vi "Begin.vi"(11 "Image Size":T1=enum."160x120") -> (0 "error out":errorcluster)   [LabVIEW 2011]
doc: "Called before other user functions, this VI is expected to open initial I/O refnums, load in file data, and do all program initialization. Notice that the <B>error out</B> terminal is simply used for data flow. Wiring it to other structures or subVIs ensures that this VI runs first."
uses:
  <vilib>/Rock Robotics/WPI/Camera/WPI_CameraImageSize.ctl
  <vilib>/Rock Robotics/WPI/Joystick/WPI_JoystickDeviceEnum.ctl
  <vilib>/Rock Robotics/WPI/Camera/WPI_CameraWhite Balance Values.ctl
  <vilib>/Rock Robotics/WPI/Camera/WPI_CameraExposure Values.ctl
  <vilib>/Rock Robotics/WPI/Camera/WPI_CameraFrameRate.ctl
  <vilib>/Rock Robotics/SystemInterfaces/DIO/FPGA_DIOPWMChannel.ctl
  <vilib>/Rock Robotics/SystemInterfaces/AI/FPGA_AIChannel.ctl
  <vilib>/Rock Robotics/WPI/MotorControl/WPI_MotorControlOpen Victor.vi
  Robot Global Data.vi
  <vilib>/Rock Robotics/WPI/RobotDrive/WPI_RobotDriveOpen4MotorWithJaguar.vi
  <vilib>/Rock Robotics/WPI/RobotDrive/WPI_RobotDriveOpen2MotorWithCANJaguar.vi
  <vilib>/Rock Robotics/WPI/RobotDrive/WPI_RobotDriveOpen4MotorWithCANJaguar.vi
  <vilib>/Rock Robotics/WPI/RobotDrive/WPI_RobotDriveOpen2MotorWithJaguar.vi
panel:
  in  "4 Moter":bool
  in  "Enable CAN":bool=TRUE
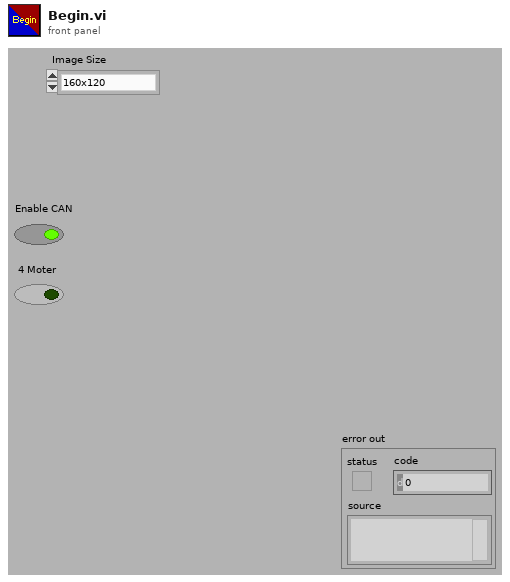
[diagram p1: front panel]
types:
  T1 = typedef "WPI_CameraImageSize.ctl" = enum16{"640x480", "320x240", "160x120"}
  T2 = typedef "FPGA_DIOPWMChannel.ctl" = enum8{"PWM 1", "PWM 2", "PWM 3", "PWM 4", "PWM 5", "PWM 6", "PWM 7", "PWM 8", "PWM 9", "PWM 10", "Invalid"}
  T3 = typedef "FPGA_AIChannel.ctl" = enum8{"AI 1", "AI 2", "AI 3", "AI 4", "AI 5", "AI 6", "AI 7", "AI 8", "Invalid"}
  T4 = typedef "WPI_JoystickDeviceEnum.ctl" = enum16{"USB 1", "USB 2", "USB 3", "USB 4", "Kinect 1", "Kinect 2"}
  T5 = typedef "WPI_CameraFrameRate.ctl" = u32
  T6 = typedef "WPI_CameraExposure Values.ctl" = enum16{"Auto", "Flicker-free 50 Hz", "Flicker-free 60 Hz", "Hold current"}
  T7 = typedef "WPI_CameraWhite Balance Values.ctl" = enum16{"Auto", "Fixed indoor", "Fixed outdoor 1", "Fixed outdoor 2", "Fixed fluorescent 1", "Fixed fluorescent 2", "Hold current"}
  T8 = typedef "WPI_JoystickDevRef.ctl" = cluster{"Device":T4}
  T9 = typedef "WPI_RobotDriveDevRef.ctl" = cluster{"DevStatus":errorcluster, "Motors[]":T10[], "Square Inputs":bool, "Max Output":dbl, "Isochronous":bool}
  T10 = typedef "WPI_MotorControlDeviceRef.ctl" = cluster{"DeviceStatus":errorcluster, "Type":enum16{"PWM", "CAN"}, "PWM":cluster{"Digital Module":T11, "PWM Channel":T2, "DeadBand":T12}, "CAN":cluster{"Device Number":u8, "Control Mode":T13, "Semaphore":T14, "Max Vout":dbl}, "Invert":bool, "TransformRef":T15, "InvTransformRef":T15}
  T11 = typedef "FPGA_TypedefDigitalModule.ctl" = enum16{"Digital Module 1", "Digital Module 2"}
  T12 = typedef "WPI_PWMDeadband.ctl" = cluster{"Name":string, "maxPositivePwm":i32, "minPositivePwm":i32, "centerPwm":i32, "maxNegativePwm":i32, "minNegativePwm":i32, "angularRange":u16}
  T13 = typedef "WPI_CANJaguar_ControlMode.ctl" = enum8{"Percent VBus", "Current", "Speed", "Position", "Voltage"}
  T14 = typedef "Semaphore RefNum" = refnum<k1>
  T15 = typedef "WPI_PWMTransform_ConPane.ctl" = refnum<vi>
  T16 = typedef "WPI_JoystickButtonState.ctl" = cluster{"Button 1":bool, "Button 2":bool, "Button 3":bool, "Button 4":bool, "Button 5":bool, "Button 6":bool, "Button 7":bool, "Button 8":bool, "Button 9":bool, "Button 10":bool, "Button 11":bool, "Button 12":bool}
  T17 = typedef "WPI_CameraDevRef.ctl" = cluster{"Camera Address":string, "CameraStatus":errorcluster, "Acquire Image Notifier":refnum<notifier>}
  T18 = enum16{"CAN Bcast - don't use", "CAN Defualt - don't use", "CAN 2 - Black Jag", "CAN 3", "CAN 4", "CAN 5", "CAN 6", "CAN 7", "CAN 8", "CAN 9"}
  T19 = typedef "WPI_AnalogChannelDevRef.ctl" = cluster{"DevStatus":errorcluster, "Analog Module":T20, "Analog Channel":T3}
  T20 = typedef "FPGA_TypedefAnalogModule.ctl" = enum16{"Analog Module 1", "Analog Module 2"}
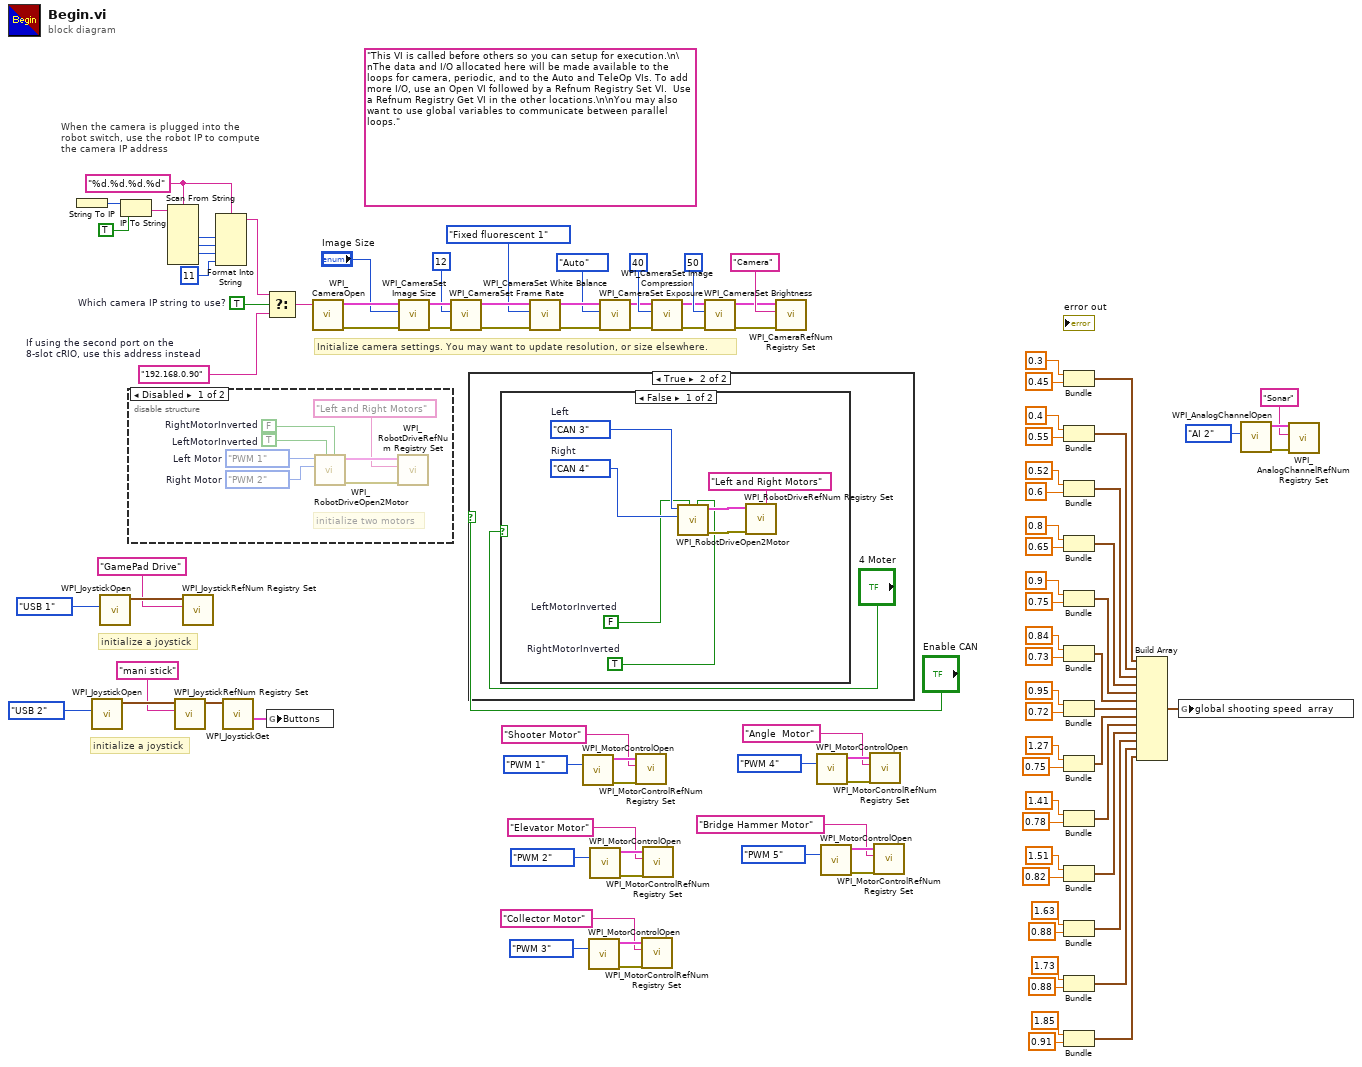
[diagram p0: block diagram]
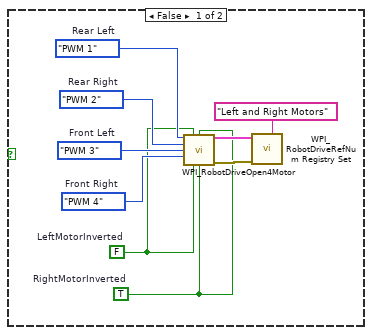
[diagram p2: hidden frame]
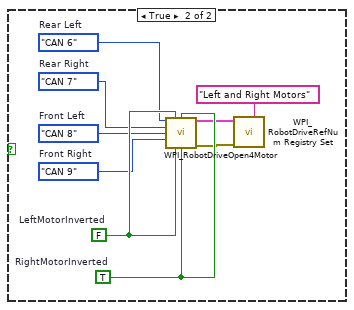
[diagram p3: hidden frame]
diagram:
  w71 = TRUE  # Which camera IP string to use?
  w75 = "%d.%d.%d.%d" ("format string")
  (unwired) "This VI is called before others so you can setup for execution.\n\nThe data and I/O allocated here will be made available to the loops for camera, periodic, and to the Auto and TeleOp VIs. To add more I/O, use an Open VI followed by a Refnum Registry Set VI.  Use a Refnum Registry Get VI in the other locations.\n\nYou may also want to use global variables to communicate between parallel loops."
  w72 = "192.168.0.90"  # If using the second port on the 8-slot cRIO, use this address instead
  # "initialize a joystick"
  # "When the camera is plugged into the\nrobot switch, use the robot IP to compute\nthe camera IP address"
  # "initialize a joystick"
  # "Initialize camera settings. You may want to update resolution, or size elsewhere."
  n1 = String To IP() -> (0:w82:u32)  [unwired: 1 in]
  n2 = call <vilib>:"WPI_JoystickOpen.vi"("JoystickDevice"=WPI_JoystickDeviceEnum."USB 2") -> ("JoystickDevRef"=w65:T8)  [unwired: 10 out]
  n3 = call <vilib>:"WPI_JoystickOpen.vi"("JoystickDevice"=WPI_JoystickDeviceEnum."USB 1") -> ("JoystickDevRef"=w105:T8)  [unwired: 10 out]
  n4 = IP To String(1:TRUE ("dot notation? (F)"), 2:w82) -> (0:w80:string)
  n5 = disable-structure shown="Disabled" {
    frame Disabled {
      w107 = FPGA_DIOPWMChannel."PWM 2"  # Right Motor
      w108 = FPGA_DIOPWMChannel."PWM 1"  # Left Motor
      w112 = TRUE  # LeftMotorInverted
      w113 = FALSE  # RightMotorInverted
      # "initialize two motors"
      n6 = call-poly <vilib>:"WPI_RobotDriveOpen2Motor.vi"("Right Motor Inverted"=w113, "Left Motor Inverted"=w112, "Right Motor"=w107, "Left Motor"=w108) -> ("error out"=w109:errorcluster, "RobotDriveDevRef"=w111:T9)  [unwired: 1 in, 5 out]
      n7 = call <vilib>:"WPI_RobotDriveRefNum Registry Set.vi"("error in (no error)"=w109, "refnum name"="Left and Right Motors", "RobotDriveDevRef"=w111) -> ()  [unwired: 9 out]
    }
    frame Enabled {
    }
  }
  n8 = Scan From String(format string=w75, input string=w80) -> (output 1=w79:i32, output 2=w78:i32, output 3=w77:i32)  [unwired: 7 in, 3 out]
  n9 = call <vilib>:"WPI_JoystickRefNum Registry Set.vi"("refnum name"="mani stick", "JoystickDevRef"=w65) -> ("JoystickDevRef"=w58:T8)  [unwired: 1 in, 8 out]
  n10 = call <vilib>:"WPI_JoystickRefNum Registry Set.vi"("refnum name"="GamePad Drive", "JoystickDevRef"=w105) -> ()  [unwired: 1 in, 9 out]
  n11 = Format Into String(format string=w75, w79, w78, w77, 11 ("Compression")) -> (resulting string=w73:string)  [unwired: 2 in, 1 out]
  n12 = call <vilib>:"WPI_JoystickGet.vi"("JoystickDevRef"=w58) -> ("Buttons"=w57:T16)  [unwired: 4 in, 2 out]
  n13 = Select(t=w73, s=w71, f=w72) -> (s? t:f=w74:string)
  n14 = global write "Robot Global Data.vi" "Buttons"(w57) -> ()
  n15 = call <vilib>:"WPI_CameraOpen.vi"("Camera Address"=w74) -> ("error out"=w95:errorcluster, "CameraDevRef"=w96:T17)  [unwired: 1 in, 8 out]
  n16 = call <vilib>:"WPI_CameraSet Image Size.vi"("error in (no error)"=w95, "Image Size"="Image Size", "CameraDevRef"=w96) -> ("error out"=w94:errorcluster, "CameraDevRef Out"=w97:T17)  [unwired: 7 out]
  n17 = call <vilib>:"WPI_CameraSet Frame Rate.vi"("error in (no error)"=w94, "Frame Rate (fps)"=T5 12, "CameraDevRef"=w97) -> ("error out"=w93:errorcluster, "CameraDevRef Out"=w99:T17)  [unwired: 7 out]
  n18 = case shown="True" "Enable CAN" {
    frame False {
      w116 = FPGA_DIOPWMChannel."PWM 4"  # Front Right
      w117 = FPGA_DIOPWMChannel."PWM 3"  # Front Left
      w118 = FPGA_DIOPWMChannel."PWM 2"  # Rear Right
      w119 = FPGA_DIOPWMChannel."PWM 1"  # Rear Left
      w115 = FALSE  # LeftMotorInverted
      w114 = TRUE  # RightMotorInverted
      n19 = call-poly <vilib>:"WPI_RobotDriveOpen4Motor.vi"("Rear Left Motor"=w119, "Rear Left Motor Inverted"=w115, "Rear Right Motor Inverted"=w114, "Rear Right Motor"=w118, "Front Left Motor"=w117, "Front Right Motor"=w116, "Front Left Motor Inverted"=w115, "Front Right Motor Inverted"=w114) -> ("RobotDriveDevRef"=w122:T9, "error out"=w120:errorcluster)  [unwired: 1 in, 5 out]
      n20 = call <vilib>:"WPI_RobotDriveRefNum Registry Set.vi"("error in (no error)"=w120, "refnum name"="Left and Right Motors", "RobotDriveDevRef"=w122) -> ()  [unwired: 9 out]
    }
    frame True {
      n21 = case shown="False" "4 Moter" {
        frame False {
          w126 = T18."CAN 4"  # Right
          w127 = T18."CAN 3"  # Left
          w125 = FALSE  # LeftMotorInverted
          w124 = TRUE  # RightMotorInverted
          n22 = call-poly <vilib>:"WPI_RobotDriveOpen2Motor.vi"("Right Motor Inverted"=w124, "Left Motor Inverted"=w125, "Right Motor"=w126, "Left Motor"=w127) -> ("error out"=w130:errorcluster, "RobotDriveDevRef"=w128:T9)  [unwired: 6 in]
          n23 = call <vilib>:"WPI_RobotDriveRefNum Registry Set.vi"("error in (no error)"=w130, "refnum name"="Left and Right Motors", "RobotDriveDevRef"=w128) -> ()  [unwired: 9 out]
        }
        frame True {
          w131 = T18."CAN 9"  # Front Right
          w132 = T18."CAN 8"  # Front Left
          w133 = T18."CAN 7"  # Rear Right
          w134 = T18."CAN 6"  # Rear Left
          w138 = FALSE  # LeftMotorInverted
          w139 = TRUE  # RightMotorInverted
          n24 = call-poly <vilib>:"WPI_RobotDriveOpen4Motor.vi"("Rear Left Motor"=w134, "Rear Left Motor Inverted"=w138, "Rear Right Motor Inverted"=w139, "Rear Right Motor"=w133, "Front Left Motor"=w132, "Front Right Motor"=w131, "Front Left Motor Inverted"=w138, "Front Right Motor Inverted"=w139) -> ("RobotDriveDevRef"=w135:T9, "error out"=w137:errorcluster)  [unwired: 1 in, 5 out]
          n25 = call <vilib>:"WPI_RobotDriveRefNum Registry Set.vi"("error in (no error)"=w137, "refnum name"="Left and Right Motors", "RobotDriveDevRef"=w135) -> ()  [unwired: 9 out]
        }
      }
    }
  }
  n26 = call <vilib>:"WPI_CameraSet White Balance.vi"("error in (no error)"=w93, "White Balance"=WPI_CameraWhite_Balance_Values."Fixed fluorescent 1", "CameraDevRef"=w99) -> ("error out"=w92:errorcluster, "CameraDevRef Out"=w98:T17)  [unwired: 7 out]
  n27 = call-poly <vilib>:"WPI_MotorControlOpen.vi"("PWM Channel"=FPGA_DIOPWMChannel."PWM 1") -> ("error out"=w69:errorcluster, "MotorControlDeviceRef"=w68:T10)  [unwired: 9 in]
  n28 = call-poly <vilib>:"WPI_MotorControlOpen.vi"("PWM Channel"=FPGA_DIOPWMChannel."PWM 3") -> ("error out"=w12:errorcluster, "MotorControlDeviceRef"=w11:T10)  [unwired: 9 in]
  n29 = call-poly <vilib>:"WPI_MotorControlOpen.vi"("PWM Channel"=FPGA_DIOPWMChannel."PWM 2") -> ("error out"=w16:errorcluster, "MotorControlDeviceRef"=w15:T10)  [unwired: 9 in]
  n30 = call <vilib>:"WPI_CameraSet Exposure.vi"("error in (no error)"=w92, "Exposure"=WPI_CameraExposure_Values."Auto", "CameraDevRef"=w98) -> ("error out"=w91:errorcluster, "CameraDevRef Out"=w101:T17)  [unwired: 7 out]
  n31 = call <vilib>:"WPI_MotorControlRefNum Registry Set.vi"("error in (no error)"=w69, "refnum name"="Shooter Motor", "MotorControlDevRef"=w68) -> ()  [unwired: 7 in, 2 out]
  n32 = call <vilib>:"WPI_MotorControlRefNum Registry Set.vi"("error in (no error)"=w12, "refnum name"="Collector Motor", "MotorControlDevRef"=w11) -> ()  [unwired: 7 in, 2 out]
  n33 = call <vilib>:"WPI_MotorControlRefNum Registry Set.vi"("error in (no error)"=w16, "refnum name"="Elevator Motor", "MotorControlDevRef"=w15) -> ()  [unwired: 7 in, 2 out]
  n34 = call <vilib>:"WPI_CameraSet Image Compression.vi"("error in (no error)"=w91, "Compression"=40, "CameraDevRef"=w101) -> ("error out"=w90:errorcluster, "CameraDevRef Out"=w100:T17)  [unwired: 7 out]
  n35 = call <vilib>:"WPI_CameraSet Brightness.vi"("error in (no error)"=w90, "Brightness"=50, "CameraDevRef"=w100) -> ("error out"=w88:errorcluster, "CameraDevRef Out"=w89:T17)  [unwired: 7 out]
  n36 = call <vilib>:"WPI_CameraRefNum Registry Set.vi"("error in (no error)"=w88, "refnum name"="Camera", "CameraDevRef"=w89) -> ()  [unwired: 9 out]
  n37 = call-poly <vilib>:"WPI_MotorControlOpen.vi"("PWM Channel"=FPGA_DIOPWMChannel."PWM 4") -> ("error out"=w8:errorcluster, "MotorControlDeviceRef"=w7:T10)  [unwired: 9 in]
  n38 = call-poly <vilib>:"WPI_MotorControlOpen.vi"("PWM Channel"=FPGA_DIOPWMChannel."PWM 5") -> ("error out"=w4:errorcluster, "MotorControlDeviceRef"=w3:T10)  [unwired: 9 in]
  n39 = call <vilib>:"WPI_MotorControlRefNum Registry Set.vi"("error in (no error)"=w8, "refnum name"="Angle  Motor", "MotorControlDevRef"=w7) -> ()  [unwired: 7 in, 2 out]
  n40 = call <vilib>:"WPI_MotorControlRefNum Registry Set.vi"("error in (no error)"=w4, "refnum name"="Bridge Hammer Motor", "MotorControlDevRef"=w3) -> ()  [unwired: 7 in, 2 out]
  n41 = Bundle(0.3, 0.45) -> (w52:cluster{dbl, dbl})  [unwired: 1 in]
  n42 = Bundle(0.4, 0.55) -> (w51:cluster{dbl, dbl})  [unwired: 1 in]
  n43 = Bundle(0.52, 0.6) -> (w42:cluster{dbl, dbl})  [unwired: 1 in]
  n44 = Bundle(0.8, 0.65) -> (w41:cluster{dbl, dbl})  [unwired: 1 in]
  n45 = Bundle(0.9, 0.75) -> (w40:cluster{dbl, dbl})  [unwired: 1 in]
  n46 = Bundle(0.84, 0.73) -> (w39:cluster{dbl, dbl})  [unwired: 1 in]
  n47 = Bundle(0.95, 0.72) -> (w30:cluster{dbl, dbl})  [unwired: 1 in]
  n48 = Bundle(1.27, 0.75) -> (w29:cluster{dbl, dbl})  [unwired: 1 in]
  n49 = Bundle(1.41, 0.78) -> (w28:cluster{dbl, dbl})  [unwired: 1 in]
  n50 = Bundle(1.51, 0.82) -> (w27:cluster{dbl, dbl})  [unwired: 1 in]
  n51 = Bundle(1.63, 0.88) -> (w23:cluster{dbl, dbl})  [unwired: 1 in]
  n52 = Bundle(1.73, 0.88) -> (w20:cluster{dbl, dbl})  [unwired: 1 in]
  n53 = Bundle(1.85, 0.91) -> (w17:cluster{dbl, dbl})  [unwired: 1 in]
  n54 = Build Array(w52, w51, w42, w41, w40, w39, w30, w29, w28, w27, w23, w20, w17) -> (w26:cluster{dbl, dbl}[])
  n55 = global write "Robot Global Data.vi" "global shooting speed  array"(w26) -> ()
  n56 = call <vilib>:"WPI_AnalogChannelOpen.vi"("Analog Channel"=FPGA_AIChannel."AI 2") -> ("error out"=w61:errorcluster, "AIDeviceRef"=w60:T19)  [unwired: 9 in]
  n57 = call <vilib>:"WPI_AnalogChannelRefNum Registry Set.vi"("error in (no error)"=w61, "refnum name"="Sonar", "AIDeviceRef"=w60) -> ()  [unwired: 7 in, 2 out]
